vi "LaserMachiningMC.vi"() -> ()   [LabVIEW 2009]
uses:
  <vilib>/Utility/SMTP/NI_SMTPEmail.lvlib
panel:
  in  "Tab Control":T1(tab)
  in  "Ring":u16(ring) items=["Machine Mode", "Write TRJs", "Do nothing"]
  in  "Pause Machining":bool
  in  "Machine this Element":bool
  in  "Create Element":bool
  in  "Make new Element":u16(ring)=5 items=["Make new Capillary", "Make new Slot", "Make new Jet", "Make new Elektrode Hole", "Create Origin Cross"]
  in  "Delete Item":bool
  in  "Element-Liste":i32[](listbox)
  in  "OK":bool
  out "Element Description":variant
  out "Element Name":string
  in  "Abort Machining":bool
  in  "Write to XPS":bool
  in  "Mail notification recipients":string[](array[string])=["ckoschitzki@lbl.gov"]
  out "Current State":string
  in  "Measured origin x,y":dbl[](array[numeric])=[0.83, 0.79]
  in  "Ture: Z home serch 2":bool
  in  "Ture: XY home serch":bool
  in  "Ture: execute trj":bool
  in  "Z Axis Position(S) (units)":dbl=13.8 format="%.6f"
  in  "Ablation Rate":dbl
  out "Move Lens":bool
  in  "XY Line Arc Trajectory":T2={"Velocity (units/s)"=2.0, "Acceleration (unts/s2)"=20.0, "Number of times of execution"=1} {"Acceleration (unts/s2)" format="%.6f"; "Velocity (units/s)" format="%.6f"; "Number of times of execution" format="%.6f"}
  in  "Group Name":string="XY"
  in  "IP address":string="192.168.0.254"
  in  "GPIO Name (DO)":string="GPIO4.DO"
  in  "SingleAxis Group  Name":string="S"
  out "error out":errorcluster
  out "XPS error out":errorcluster
  out "XPS error out(FTP put)":errorcluster
  out "invalid recipients":string[](array[string])
  out "connection ID out":T3
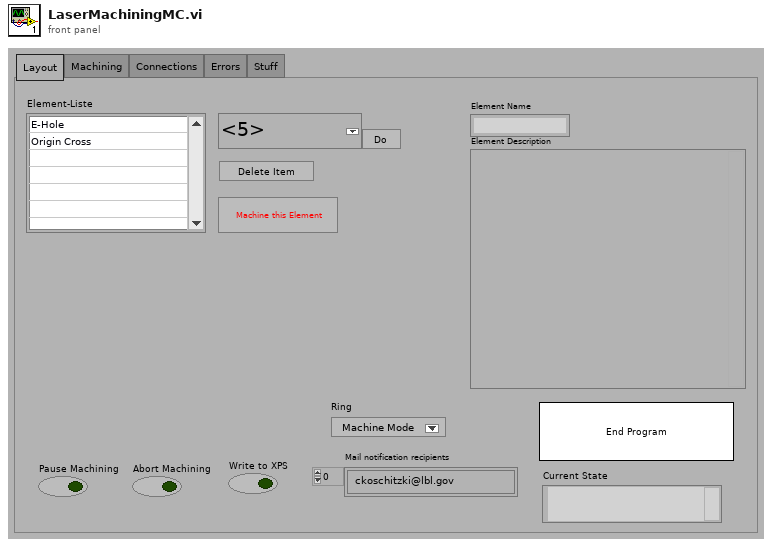
[diagram p1: front panel]
types:
  T1 = enum32{"Layout", "Machining", "Connections", "Errors", "Stuff"}
  T2 = cluster{"Velocity (units/s)":dbl, "Acceleration (unts/s2)":dbl, "Number of times of execution":i32}
  T3 = cluster{"connection TCP":refnum<k5>, "LogTo File":bool, "Log File refnum":refnum<file>, "no error if error log":bool}
  T4 = enum32{"invalid app kind", "Development System", "Run Time System", "Student Edition", "Embedded LabVIEW", "Evaluation", "Custom"}
  T5 = enum32{"Invalid", "Standard", "Closed", "Hidden", "Minimized", "Maximized"}
  T6 = cluster{"Core":cluster{"Current VI Reference":refnum<vi>, "Close Panel on Exit?":bool}, "Elements List":cluster{"Element name":string, "Type":i32, "Layer per L-Move":i32, "Variant":variant}[], "Elements available":cluster{"path":path, "Elements Name":string, "Type":i32}[], "TRJ Cluster":cluster{"TRJs":path[], "size(s)":i32, "Start Point":dbl[][]}, "Start Point":dbl[][], "Additional Stuff":i32, "connection ID":cluster{"connection TCP":refnum<k5>, "LogTo File":bool, "Log File refnum":refnum<file>, "no error if error log":bool}, "IP address":string, "Current TRJ":i32, "GPIO Name (DO) ":string, "XPS error":errorcluster, "Group Name":string, "Measured origin x,y":dbl[], "XY Line Arc Trajectory":cluster{"Velocity (units/s)":dbl, "Acceleration (unts/s2)":dbl, "Number of times of execution":i32}, "Actual Element":cluster{"Element name":string, "Type":i32, "Layer per L-Move":i32, "Variant":variant}}
  T7 = cluster{"Element name":string, "Type":i32, "Layer per L-Move":i32, "Variant":variant}[]
  T8 = cluster{"Element name":string, "Type":i32, "Layer per L-Move":i32, "Variant":variant}
  T9 = cluster{"TRJs":path[], "size(s)":i32, "Start Point":dbl[][]}
  T10 = cluster{"Current VI Reference":refnum<vi>, "Close Panel on Exit?":bool}
  T11 = cluster{"path":path, "Elements Name":string, "Type":i32}[]
  T12 = cluster{"path":path, "Elements Name":string, "Type":i32}
  T13 = cluster{"trj file path(1)":path[], "size(s)":i32, dbl[][]}
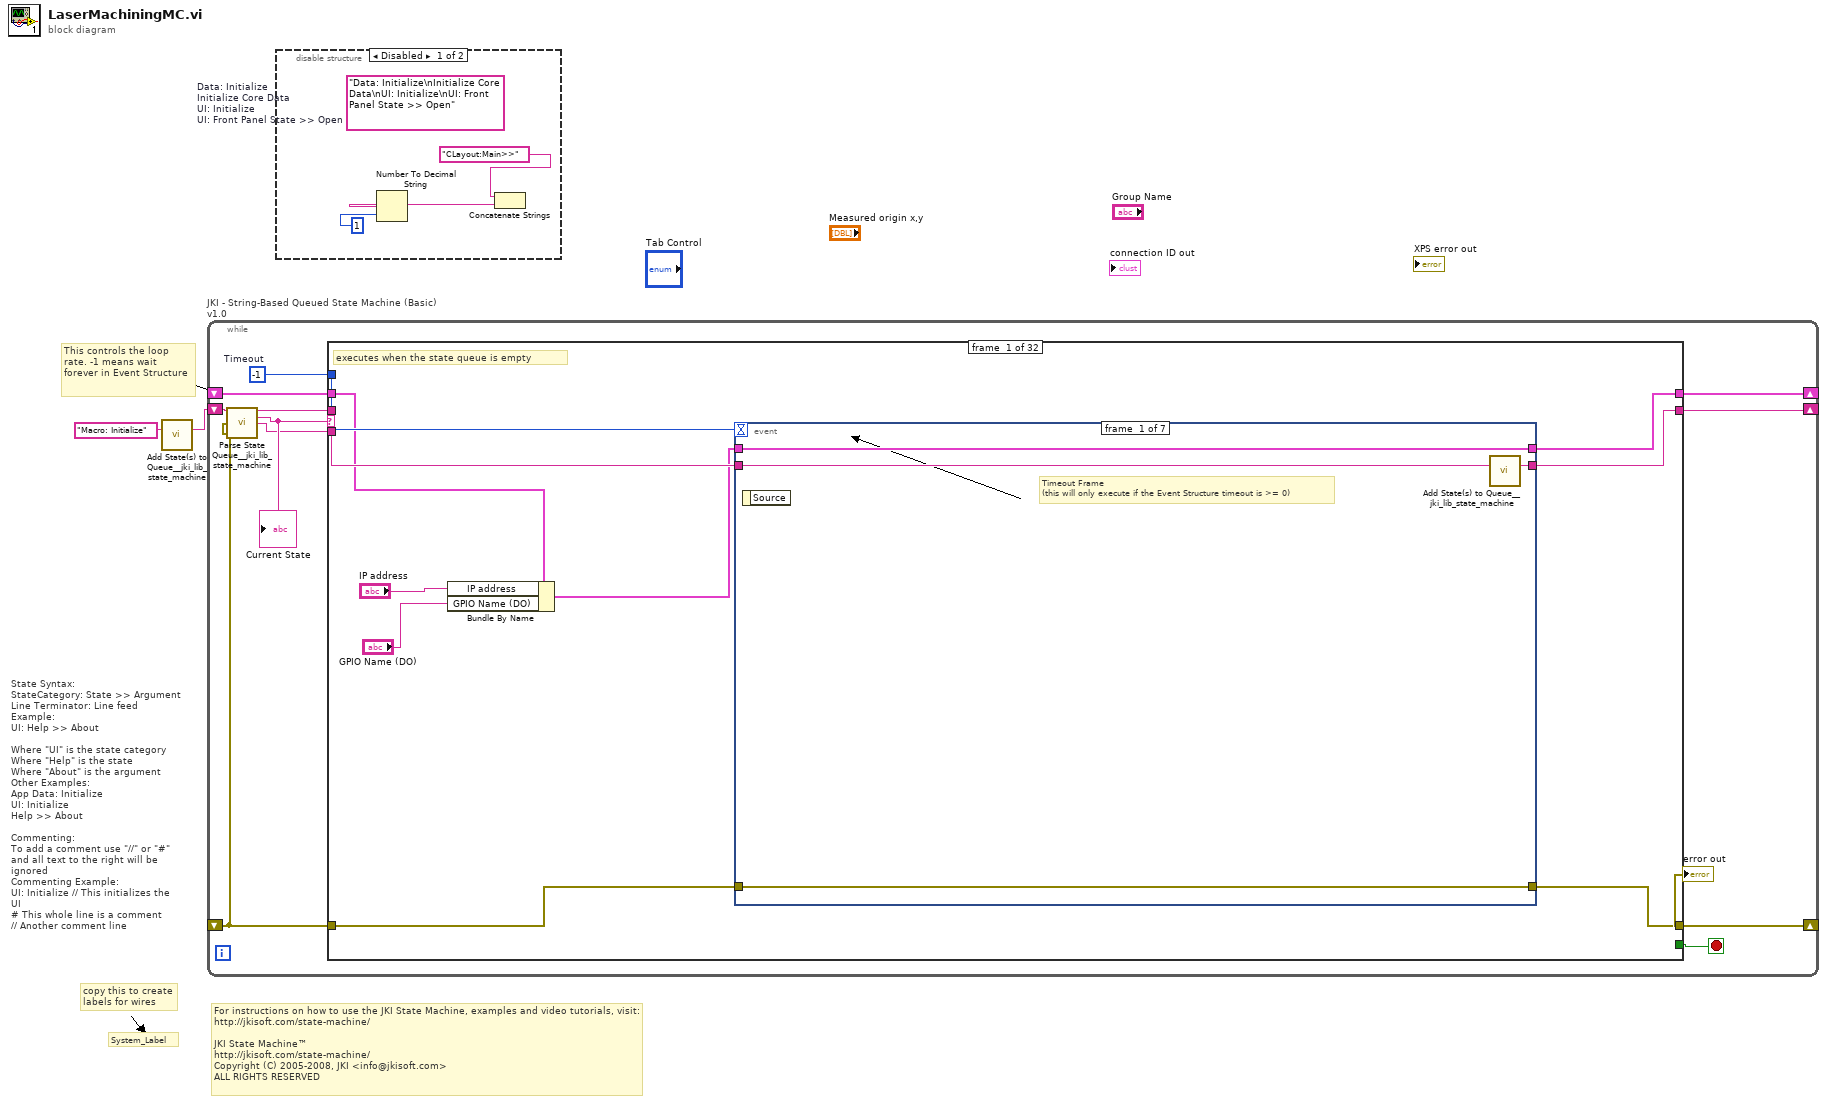
[diagram p0: block diagram]
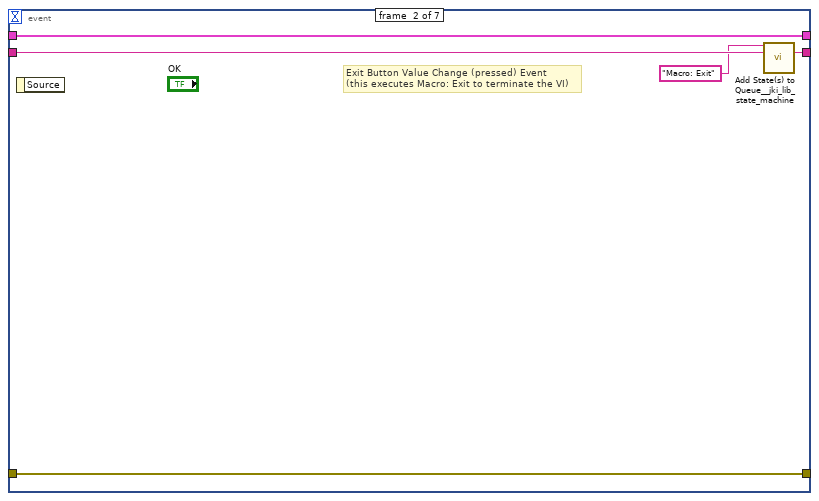
[diagram p3: hidden frame]
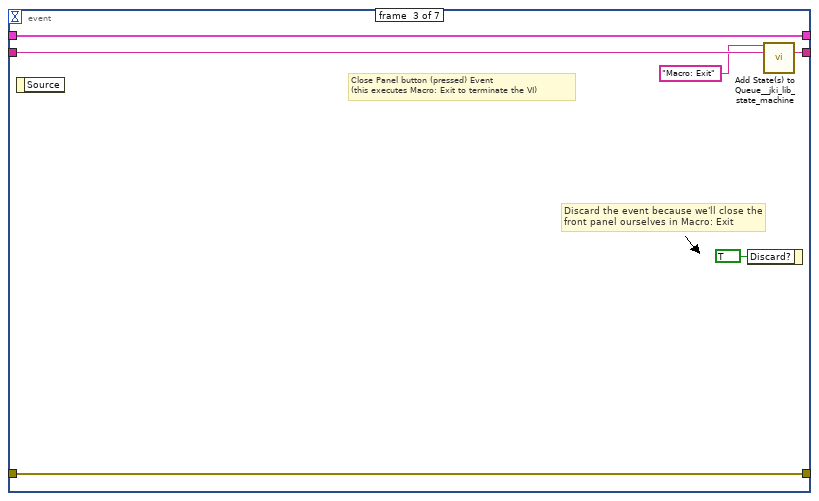
[diagram p4: hidden frame]
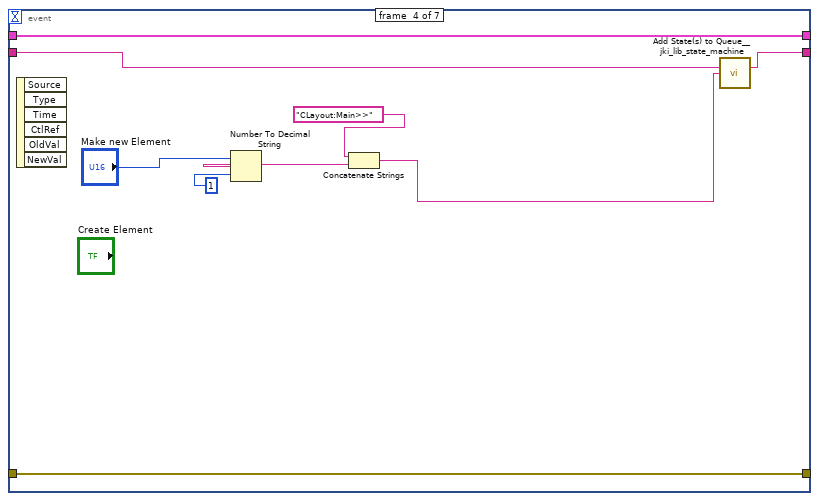
[diagram p5: hidden frame]
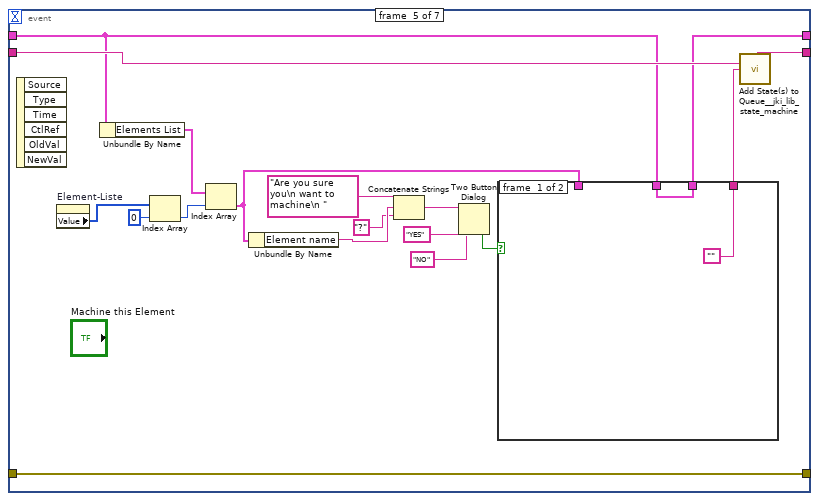
[diagram p6: hidden frame]
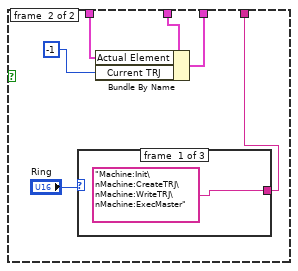
[diagram p7: hidden frame]
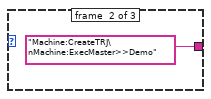
[diagram p8: hidden frame]
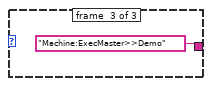
[diagram p9: hidden frame]
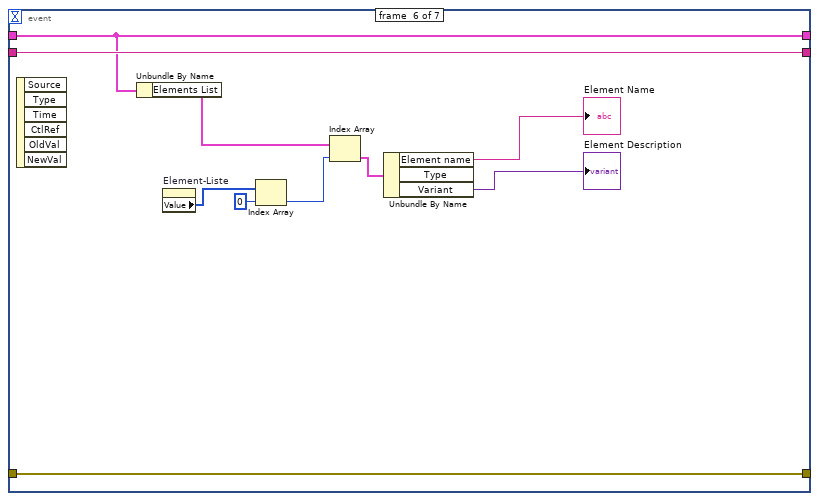
[diagram p10: hidden frame]
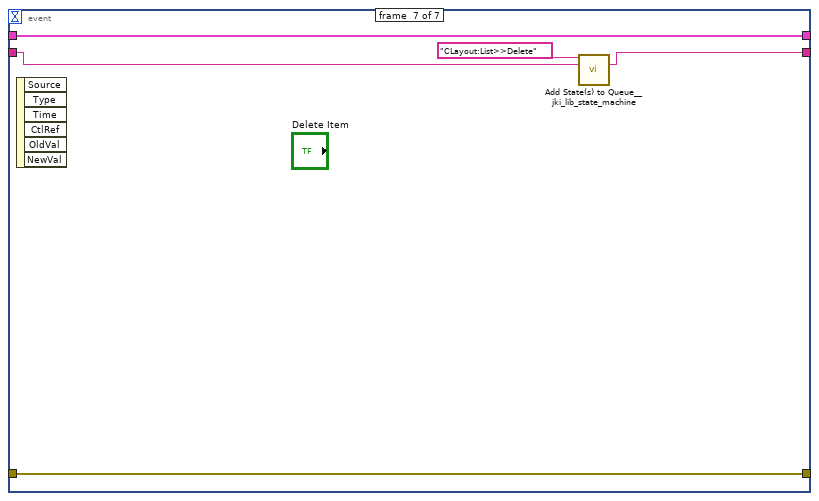
[diagram p11: hidden frame]
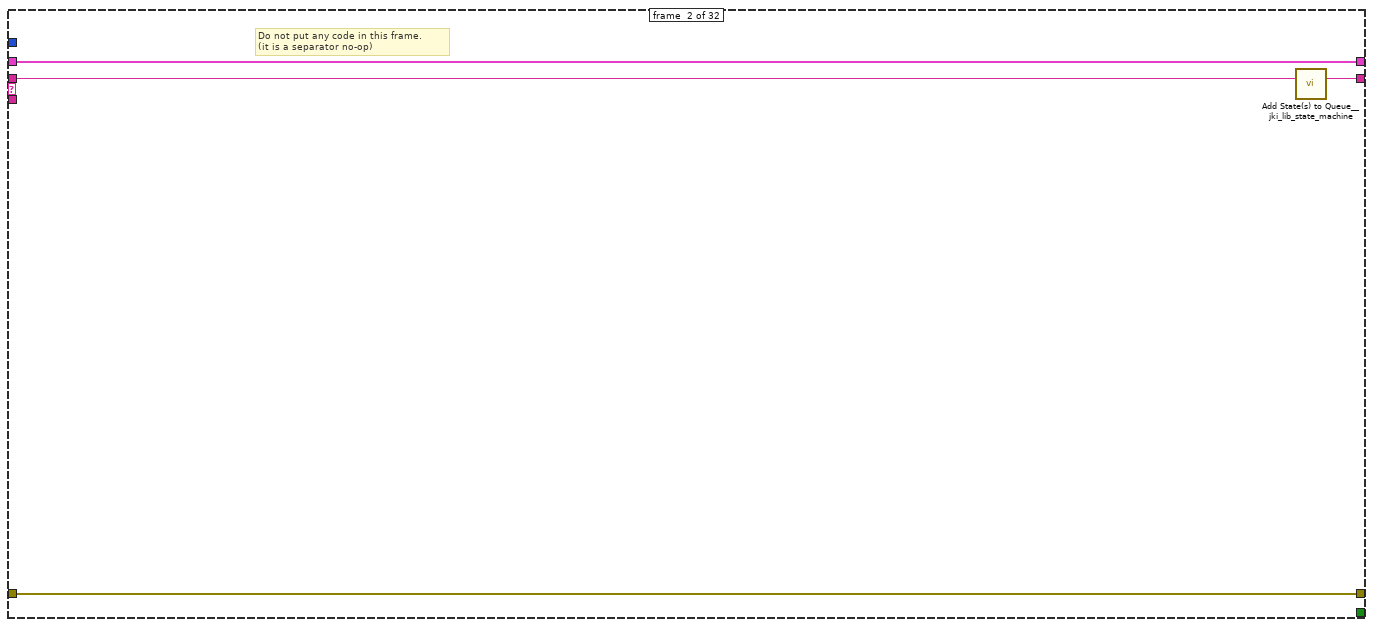
[diagram p12: hidden frame]
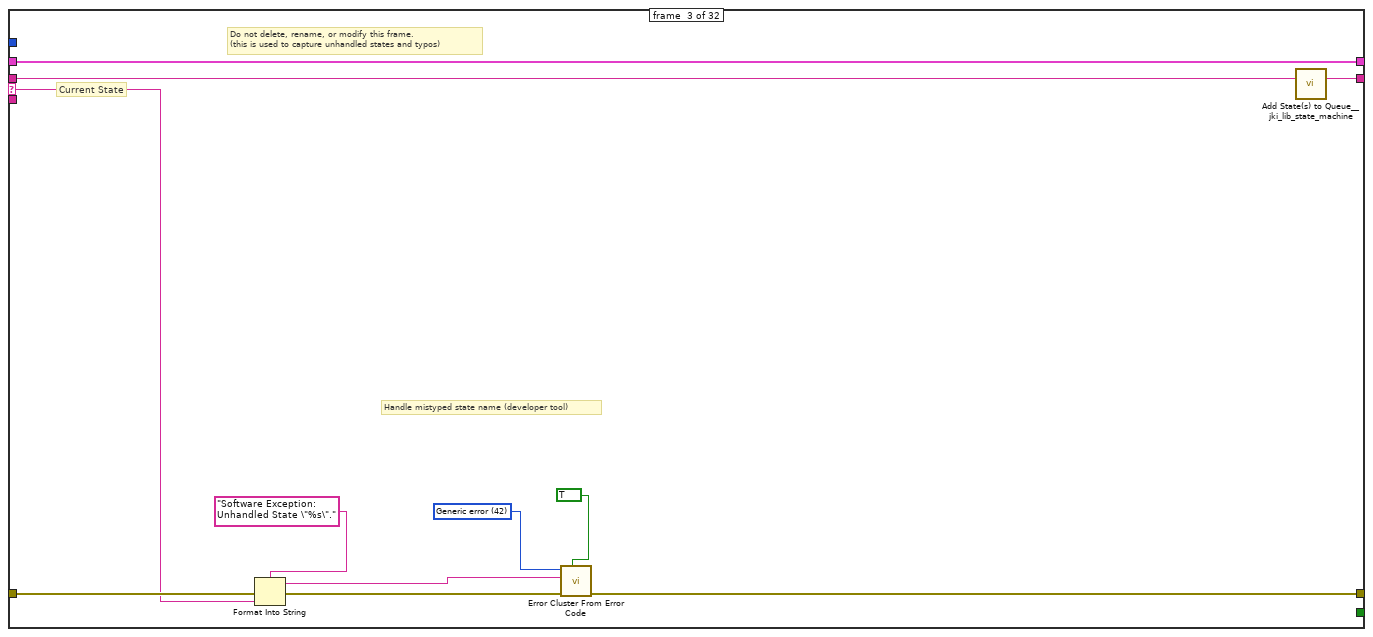
[diagram p13: hidden frame]
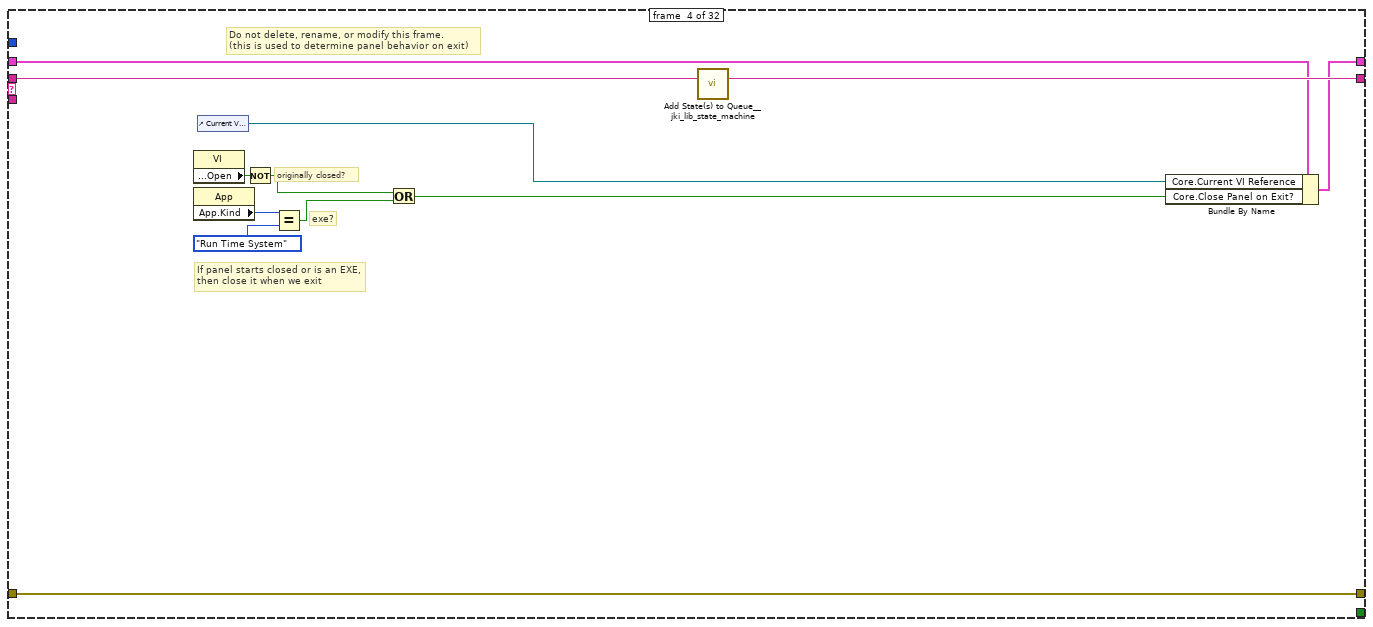
[diagram p14: hidden frame]
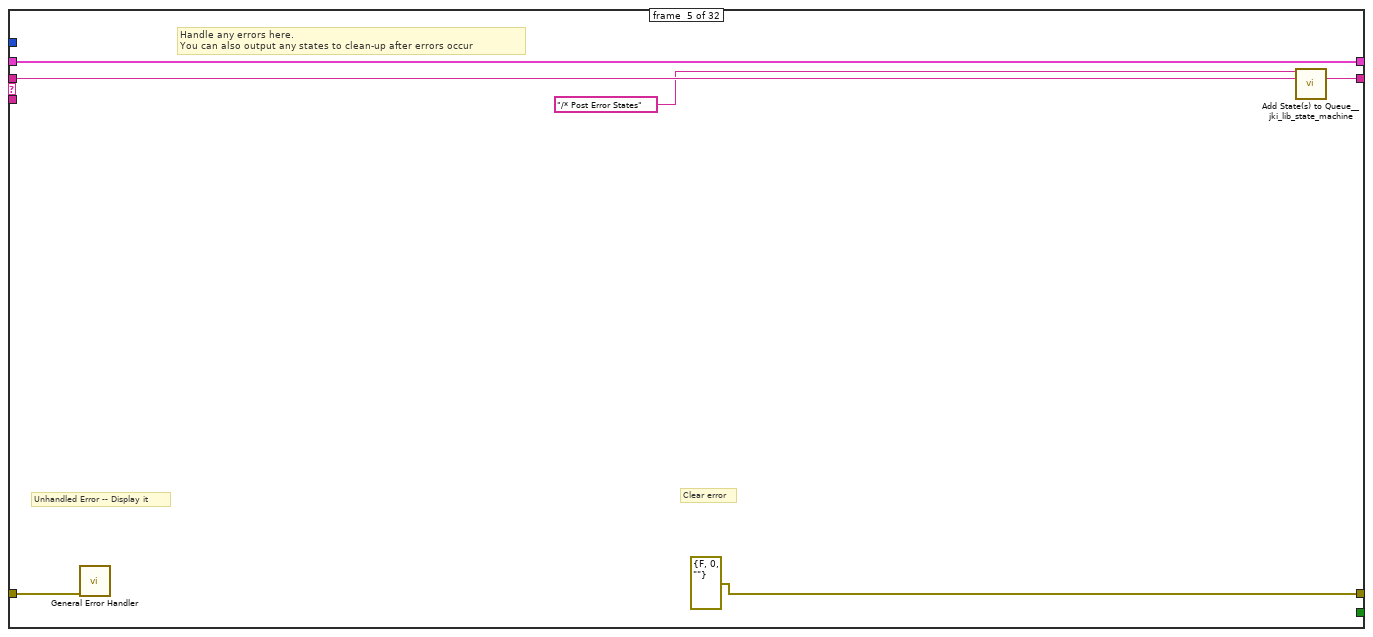
[diagram p15: hidden frame]
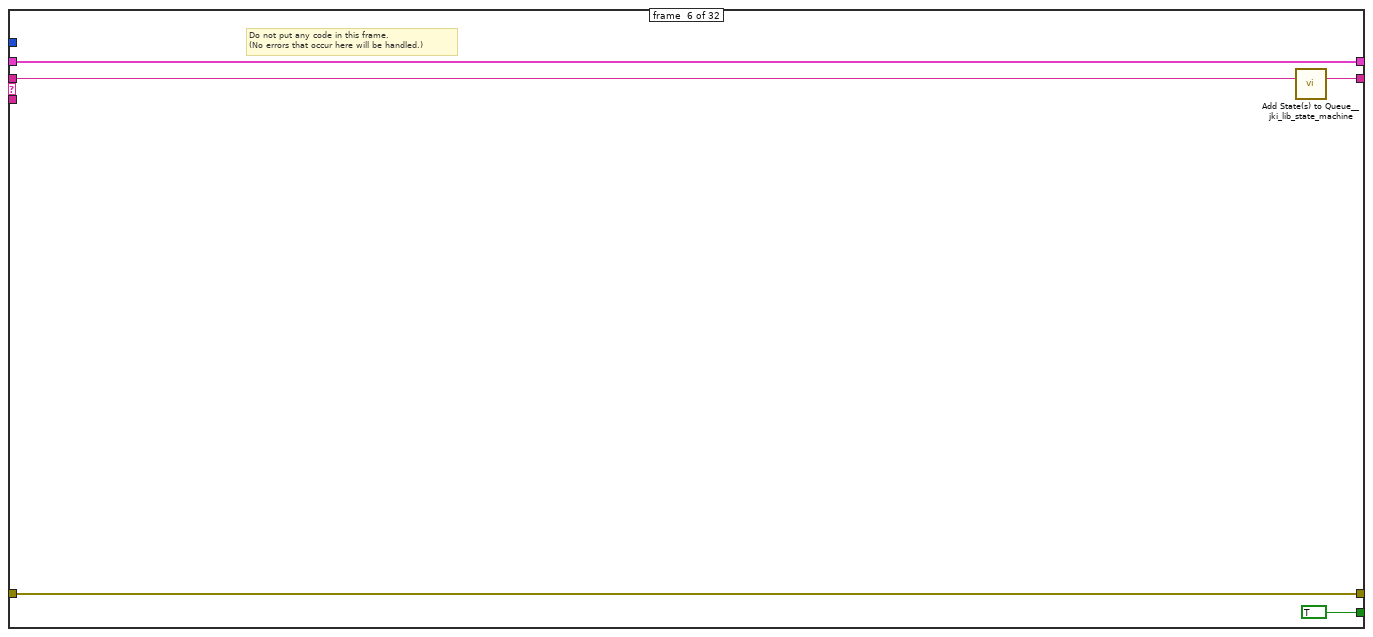
[diagram p16: hidden frame]
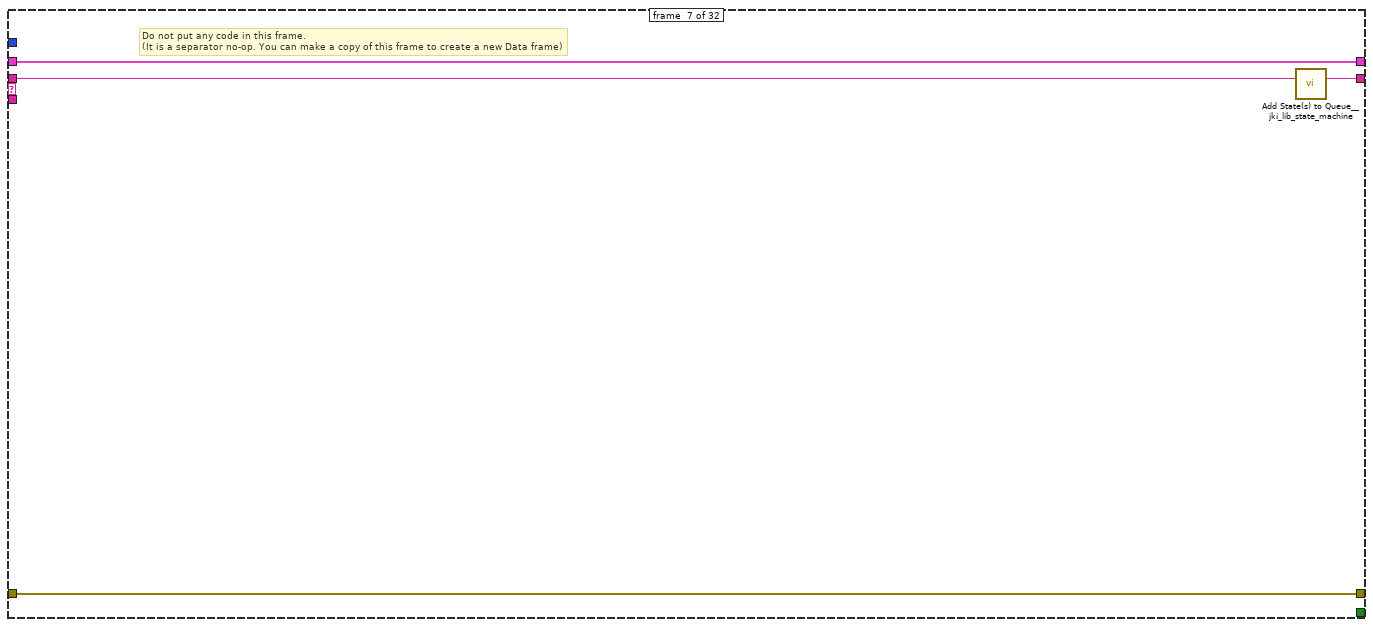
[diagram p17: hidden frame]
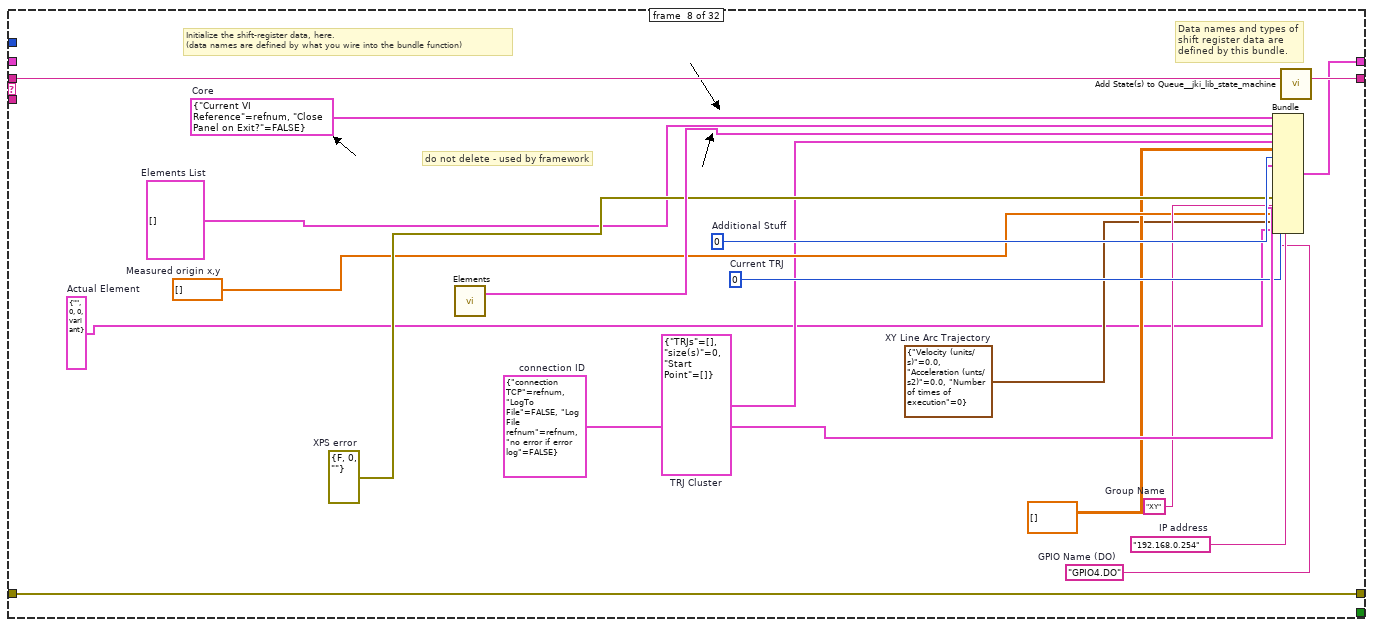
[diagram p18: hidden frame]
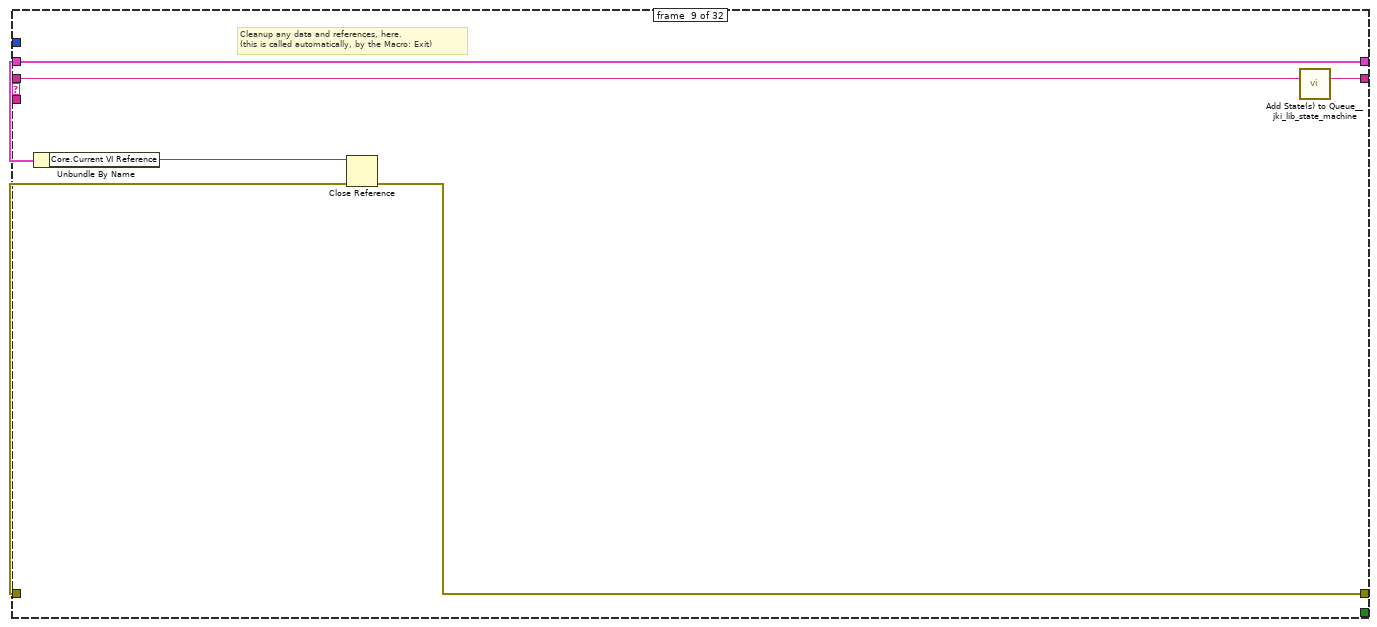
[diagram p19: hidden frame]
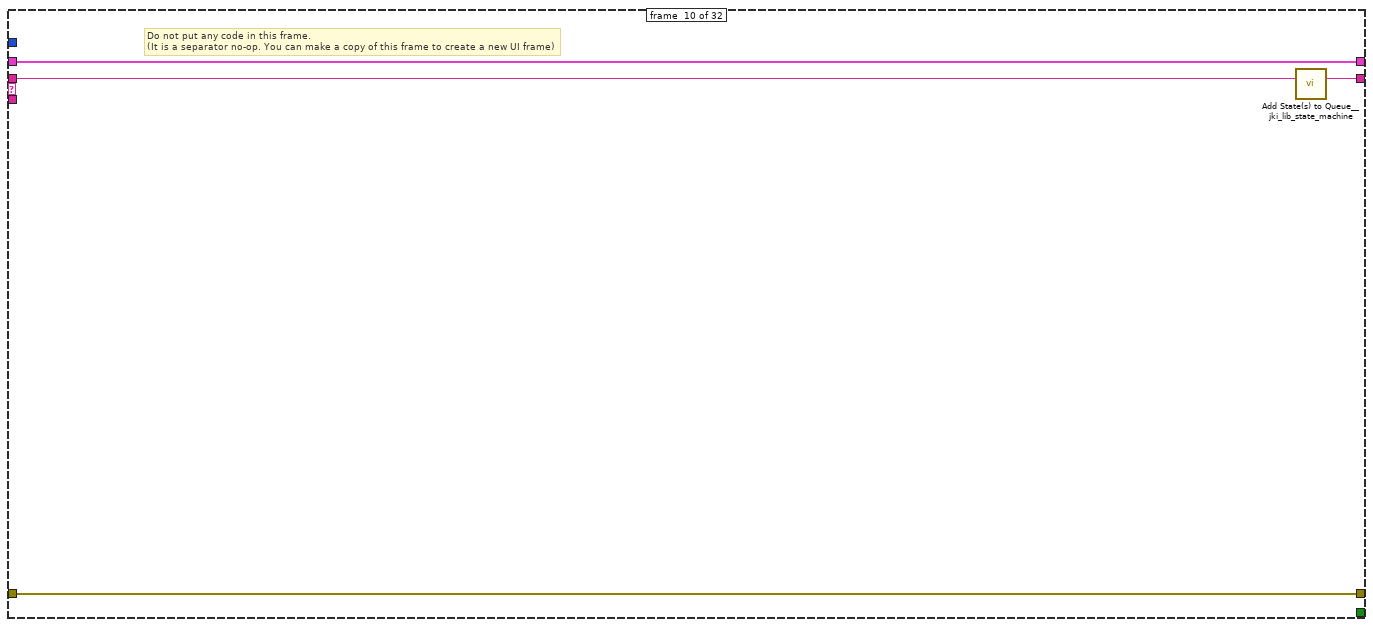
[diagram p20: hidden frame]
diagram:
  # "For instructions on how to use the JKI State Machine, examples and video tutorials, visit:\nhttp://jkisoft.com/state-machine/\n\nJKI State Machine™\nhttp://jkisoft.com/state-machine/\nCopyright (C) 2005-2008, JKI <info@jkisoft.com>\nALL RIGHTS RESERVED"
  # "State Syntax:\nStateCategory: State >> Argument\nLine Terminator: Line feed\nExample:\nUI: Help >> About\n\nWhere \"UI\" is the state category\nWhere \"Help\" is the state\nWhere \"About\" is the argument\nOther Examples:\nApp Data: Initialize\nUI: Initialize\nHelp >> About\n\nCommenting:\nTo add a comment use \"//\" or \"#\" and all text to the right will be ignored\nCommenting Example:\nUI: Initialize // This initializes the UI\n# This whole line is a comment\n// Another comment line"
  # "copy this to create labels for wires"
  # "This controls the loop rate. -1 means wait forever in Event Structure"
  # "System_Label"
  n1 = call <vilib>:"Add State(s) to Queue__jki_lib_state_machine.vi"("State(s) in (\"\")"="Macro: Initialize") -> ("States Out"=w2:string)  [unwired: 14 in]
  n2 = while "JKI - String-Based Queued State Machine (Basic) v1.0" {
    shift-right: [w4] -> _
    shift-left: _ -> [w7]
    shift-right: [w3] -> _
    shift-left: _ -> [w5]
    shift-right: [w9] -> _
    shift-left: w2 -> [w10]
    stop <- w8 stop-if-true
    w6 = -1  # Timeout
    # "Template Copyright © 2008 JKI - http://jkisoft.com/state-machine"
    n3 = call <vilib>:"Parse State Queue__jki_lib_state_machine.vi"("State Queue"=w10, "Error In (no error)"=w5) -> ("Remaining States"=w12:string, "Current State"=w13:string, "Arguments"=w11:string)  [unwired: 11 in]
    "Current State" <- w13
    n4 = case shown="\"CLayout:Main\"" w13 {
      selector: w13 -> [_ _ w96 _ _ _ _ _ _ _ _ _ _ _ _ _ _ _ _ _ _ _ _ _ _ _ _ _ _ _ _ _]
      tunnel: w12 -> [w23 w95 w100 w118 w124 w129 w133 w152 w158 w162 w172 w178 w189 w213 w218 w228 w232 w235 w270 w307 w319 w334 w349 w426 w433 w489 w504 w531 w532 w558 w579 w586]
      tunnel: w11 -> [_ _ _ _ _ _ _ _ _ _ _ w173 w184 _ _ _ _ w236 w265 _ w313 _ w335 _ _ w492 _ _ w539 _ _ _]
      tunnel: w7 -> [w17 w92 w98 w108 w121 w127 w130 _ w154 w159 w169 w176 w183 w210 w215 w219 w229 w238 w264 w304 w317 w331 w339 w424 w431 w490 w505 w528 w537 w557 w578 w583]
      tunnel: [w21 w93 w102 w116 errorcluster {"status"=FALSE, "code"=0, "source"=""} ("error out") w126 w131 w150 w155 w160 w163 w174 w186 w211 w216 w226 w230 w237 w267 w305 w311 w332 w347 w408 w435 w487 w501 w529 w540 w549 w580 w584] -> w3
      tunnel: w5 -> [w20 w93 w101 w116 w120 w126 w131 w150 w156 w160 w166 w175 w187 w211 w216 w226 w230 w237 w268 w305 w312 w332 w347 w409 w438 w488 w502 w530 w541 w550 w581 w584]
      tunnel: [w22 w94 w99 w117 w123 w128 w132 w151 w157 w161 w171 w177 w188 w212 w217 w227 w231 w234 w269 w306 w318 w333 w348 w426 w433 w489 w504 w531 w532 w558 w579 w585] -> w9
      tunnel: [_ _ _ _ _ TRUE _ _ _ _ _ _ _ _ _ _ _ _ _ _ _ _ _ _ _ _ _ _ _ _ _ _] -> w8
      tunnel: [w19 w92 w98 w107 w121 w127 w130 w148 w154 w159 w169 w176 w183 w210 w215 w219 w229 w233 w266 w304 w317 w331 w338 w425 w429 w490 w505 w527 w533 w555 w578 w583] -> w4
      tunnel: w6 -> [w18 _ _ _ _ _ _ _ _ _ _ _ _ _ _ _ _ _ _ _ _ _ _ _ _ _ _ _ _ _ _ _]
      frame #0 {
        # "executes when the state queue is empty"
        n5 = Bundle By Name(cluster=w17, "IP address"="IP address", "GPIO Name (DO)"="GPIO Name (DO)") -> (w16:T6)
        n6 = event shown="[4] \"Machine this Element\": Value Change" {
          selector: _ -> [_ _ _ _ _ _ _]
          dyn-events: _ -> [_ _ _ _ _ _ _]
          timeout: w18 -> [_ _ _ _ _ _ _]
          tunnel: w23 -> [w27 w32 w38 w46 w64 w86 w90]
          tunnel: [w26 w31 w37 w45 w63 w86 w89] -> w22
          tunnel: w16 -> [w24 w29 w35 w40 w51 w85 w91]
          tunnel: [w25 w30 w36 w47 w65 w84 w87] -> w21
          tunnel: w20 -> [w25 w30 w36 w47 w65 w84 w87]
          tunnel: [w24 w29 w35 w40 w50 w85 w91] -> w19
          event #0 {
            # "Timeout Frame\n(this will only execute if the Event Structure timeout is >= 0)"
            n7 = event-data() -> ()  [unwired: 1 in, 1 out]
            n8 = call <vilib>:"Add State(s) to Queue__jki_lib_state_machine.vi"("State(s) in (\"\")"=w27) -> ("States Out"=w26:string)  [unwired: 14 in]
          }
          event #1 {
            # "Exit Button Value Change (pressed) Event\n(this executes Macro: Exit to terminate the VI)"
            n9 = event-data() -> ()  [unwired: 1 in, 1 out]
            n10 = call <vilib>:"Add State(s) to Queue__jki_lib_state_machine.vi"("State(s) in Front (\"\")"="Macro: Exit", "State(s) in (\"\")"=w32) -> ("States Out"=w31:string)  [unwired: 13 in]
          }
          event #2 {
            # "Discard the event because we'll close the front panel ourselves in Macro: Exit"
            # "Close Panel button (pressed) Event\n(this executes Macro: Exit to terminate the VI)"
            n11 = event-data() -> ()  [unwired: 1 in, 1 out]
            n12 = event-data("Discard?"=TRUE) -> ()  [unwired: 1 in, 1 out]
            n13 = call <vilib>:"Add State(s) to Queue__jki_lib_state_machine.vi"("State(s) in Front (\"\")"="Macro: Exit", "State(s) in (\"\")"=w38) -> ("States Out"=w37:string)  [unwired: 13 in]
          }
          event #3 {
            n14 = event-data() -> ()  [unwired: 1 in, 6 out]
            n15 = Number To Decimal String(number="Make new Element", width (-)=i16 1) -> (decimal integer string=w42:string)
            n16 = Concatenate Strings("CLayout:Main>>" ("State(s) in Front (\"\")"), w42) -> (w39:string)
            n17 = call <vilib>:"Add State(s) to Queue__jki_lib_state_machine.vi"("State(s) in (\"\")"=w46, "State(s) at Back (\"\")"=w39) -> ("States Out"=w45:string)  [unwired: 13 in]
          }
          event #4 {
            n18 = event-data() -> ()  [unwired: 1 in, 6 out]
            n19 = property on="Element-Liste" class="LstBox (strict)"() -> ("Value"=w62:i32[])  [unwired: 2 in, 2 out]
            n20 = Unbundle By Name(w51) -> ("Elements List"=w60:T7)
            n21 = Index Array(array=w62, index=0) -> (element=w59:i32)
            n22 = Index Array(array=w60, index=w59) -> (element=w49:T8)
            n23 = Unbundle By Name(w49) -> ("Element name"=w58:string)
            n24 = Concatenate Strings("Are you sure you\n want to machine\n " ("message"), w58, "?" ("string")) -> (w56:string)
            n25 = Two Button Dialog(message=w56, 1:"NO" ("F button name (\"Cancel\")"), 2:"YES" ("T button name (\"OK\")")) -> (T button?=w52:bool)
            n26 = case shown="True" w52 {
              tunnel: w51 -> [w67 w73]
              tunnel: [w67 w72] -> w50
              tunnel: w49 -> [_ w71]
              tunnel: ["" w68] -> w48
              frame #0 {
              }
              frame #1 {
                n27 = case shown="1" "Ring" {
                  tunnel: ["Machine:Init\nMachine:CreateTRJ\nMachine:WriteTRJ\nMachine:ExecMaster" ("message") "Machine:CreateTRJ\nMachine:ExecMaster>>Demo" ("message") "Machine:ExecMaster>>Demo" ("message")] -> w68
                  frame #0 {
                  }
                  frame #1 {
                  }
                  frame #2 {
                  }
                }
                n28 = Bundle By Name(cluster=w73, "Actual Element"=w71, "Current TRJ"=-1) -> (w72:T6)
              }
            }
            n29 = call <vilib>:"Add State(s) to Queue__jki_lib_state_machine.vi"("State(s) in (\"\")"=w64, "State(s) at Back (\"\")"=w48) -> ("States Out"=w63:string)  [unwired: 13 in]
          }
          event #5 {
            n30 = event-data() -> ()  [unwired: 1 in, 6 out]
            n31 = Unbundle By Name(w85) -> ("Elements List"=w80:T7)
            n32 = property on="Element-Liste" class="LstBox (strict)"() -> ("Value"=w83:i32[])  [unwired: 2 in, 2 out]
            n33 = Index Array(array=w83, index=0) -> (element=w81:i32)
            n34 = Index Array(array=w80, index=w81) -> (element=w79:T8)
            n35 = Unbundle By Name(w79) -> ("Element name"=→"Element Name":string, "Variant"=→"Element Description":variant)  [unwired: 1 out]
          }
          event #6 {
            n36 = event-data() -> ()  [unwired: 1 in, 6 out]
            n37 = call <vilib>:"Add State(s) to Queue__jki_lib_state_machine.vi"("State(s) in Front (\"\")"="CLayout:List>>Delete" ("State(s) in Front (\"\")"), "State(s) in (\"\")"=w90) -> ("States Out"=w89:string)  [unwired: 13 in]
          }
        }
      }
      frame #1 {
        # "Do not put any code in this frame.\n(it is a separator no-op)"
        n38 = call <vilib>:"Add State(s) to Queue__jki_lib_state_machine.vi"("State(s) in (\"\")"=w95) -> ("States Out"=w94:string)  [unwired: 14 in]
      }
      frame #2 {
        w105 = 42 items=["No error", "Argument error", "Memory is full", "Out of zone", "End of file", "File already open", "Generic file I/O error", "File not found", "File permission error", "Disk is full", "Duplicate path", "Too many files open", "System feature not enabled", "Resource file not found", "Cannot add resource", "Resource not found", "Image not found", "Image memory error", "Pen does not exist", "Config type invalid", "Config token not found", "Config parse error", "Config memory error", "Bad external code format", "Bad external code offset", "External code not present", "Null window", "Destroy window error", "Null menu", "Print aborted", "Bad print record", "Print driver error", "Windows error during printing", "Memory error during printing", "Print dialog error", "Generic print error", "Invalid device refnum", "Device not found", "Device parameter error", "Device unit error", "Cannot open device", "Device call aborted", "Generic error", "Cancelled by user", "Object ID too low", "Object ID too high", "Object not in heap", "Unknown heap", "Unknown object (invalid DefProc)", "Unknown object (DefProc not in table)", "Message out of range", "Invalid (null) method", "Unknown message", "Manager call not supported", "Bad address", "Network operation in progress", "Network operation timed out", "Connection is busy", "Network attribute not supported", "Network error", "Address in use", "System out of memory", "Connection aborted", "Connection refused", "Not connected", "Already connected", "Connection closed", "Initialization error (interapplication manager)", "Bad occurrence", "Wait on unbound occurrence handler", "Occurrence queue overflow", "Datalog type conflict", "Unused", "Unrecognized type (interapplication manager)", "Memory corrupt", "Failed to make temporary DLL", "Old CIN version", "Drag socket not found", "Failed to load drop-object", "Failed to register OLE object", "Failed to release OLE object", "Format specifier type mismatch", "Unknown format specifier", "Too few format specifiers", "Too many format specifiers", "Scan failed", "Newer CIN version", "Error converting to variant", "Runtime menu error", "Password tampered", "Variant attribute not found", "Incompatible variant data type", "Event data is not available", "Event Store is not present", "Occurrence is not found", "Event Queue is not created", "Event info is not available", "Refnum passed is NULL", "Error retrieving Class GUID", "Error retrieving CoClass GUID", "Error retrieving TypeLib GUID.", "Bad built application magic bytes.", "Specific driver is different from the specific driver associated with the Logical Name.", "There is no session opened to the class driver.", "Max Error", "MAX - Error with config objects", "MAX - Error loading configuration", "MAX - Group not supported"]
        # "Current State"
        # "Do not delete, rename, or modify this frame.\n(this is used to capture unhandled states and typos)"
        # "Handle mistyped state name (developer tool)"
        n39 = Format Into String(format string="Software Exception: Unhandled State \"%s\"." ("message"), error in=w101, w96) -> (resulting string=w104:string, error out=w103:errorcluster)  [unwired: 1 in]
        n40 = call <vilib>:"Error Cluster From Error Code.vi"("show call chain? (False)"=TRUE, "error in (no error)"=w103, "error message (\"\")"=w104, "error code (0)"=w105) -> ("error out"=w102:errorcluster)  [unwired: 5 in]
        n41 = call <vilib>:"Add State(s) to Queue__jki_lib_state_machine.vi"("State(s) in (\"\")"=w100) -> ("States Out"=w99:string)  [unwired: 14 in]
      }
      frame #3 {
        # "Do not delete, rename, or modify this frame.\n(this is used to determine panel behavior on exit)"
        # "originally closed?"
        # "exe?"
        # "If panel starts closed or is an EXE, then close it when we exit"
        n42 = property class="VI"() -> ("Front Panel.Open"=w115:bool)  [unwired: 2 in, 2 out]
        n43 = property class="App"() -> ("App.Kind"=w114:T4)  [unwired: 2 in, 2 out]
        n44 = control-ref of="Current VI Reference"() -> (w109:refnum<vi>)
        n45 = Not(x=w115) -> (.not. x?=w112:bool)
        n46 = Equal?(x=w114, y=T4."Run Time System" ("Application:Kind")) -> (x = y?=w111:bool)
        n47 = Or(x=w112, y=w111) -> (x .or. y?=w110:bool)
        n48 = call <vilib>:"Add State(s) to Queue__jki_lib_state_machine.vi"("State(s) in (\"\")"=w118) -> ("States Out"=w117:string)  [unwired: 14 in]
        n49 = Bundle By Name(cluster=w108, "Core.Current VI Reference"=w109, "Core.Close Panel on Exit?"=w110) -> (w107:T6)
      }
      frame #4 {
        # "Unhandled Error -- Display it"
        # "Handle any errors here.\nYou can also output any states to clean-up after errors occur"
        # "Clear error"
        n50 = call <vilib>:"General Error Handler.vi"("error in (no error)"=w120) -> ()  [unwired: 10 in, 5 out]
        n51 = call <vilib>:"Add State(s) to Queue__jki_lib_state_machine.vi"("State(s) in Front (\"\")"="/* Post Error States", "State(s) in (\"\")"=w124) -> ("States Out"=w123:string)  [unwired: 13 in]
      }
      frame #5 {
        # "Do not put any code in this frame.\n(No errors that occur here will be handled.)"
        n52 = call <vilib>:"Add State(s) to Queue__jki_lib_state_machine.vi"("State(s) in (\"\")"=w129) -> ("States Out"=w128:string)  [unwired: 14 in]
      }
      frame #6 {
        # "Do not put any code in this frame.\n(It is a separator no-op. You can make a copy of this frame to create a new Data frame)"
        n53 = call <vilib>:"Add State(s) to Queue__jki_lib_state_machine.vi"("State(s) in (\"\")"=w133) -> ("States Out"=w132:string)  [unwired: 14 in]
      }
      frame #7 {
        w134 = T8 {"Element name"="", "Type"=0, "Layer per L-Move"=0, "Variant"=variant}  # Actual Element
        w135 = T7 []  # Elements List
        w136 = T2 {"Velocity (units/s)"=0.0, "Acceleration (unts/s2)"=0.0, "Number of times of execution"=0}  # XY Line Arc Trajectory
        w137 = T9 {"TRJs"=[], "size(s)"=0, "Start Point"=[]}  # TRJ Cluster
        w139 = dbl[] []  # Measured origin x,y
        w140 = "XY"  # Group Name
        w141 = errorcluster {"status"=FALSE, "code"=0, "source"=""}  # XPS error
        w142 = "GPIO4.DO"  # GPIO Name (DO)
        w143 = 0  # Current TRJ
        w144 = "192.168.0.254"  # IP address
        w145 = T3 {"connection TCP"=refnum, "LogTo File"=FALSE, "Log File refnum"=refnum, "no error if error log"=FALSE}  # connection ID
        w146 = 0  # Additional Stuff
        w149 = T10 {"Current VI Reference"=refnum, "Close Panel on Exit?"=FALSE}  # Core
        # "do not delete - used by framework"
        # "Data names and types of shift register data are defined by this bundle."
        # "Initialize the shift-register data, here.\n(data names are defined by what you wire into the bundle function)"
        n54 = call "Elements.vi"() -> ("Elements available"=w147:T11)  [unwired: 2 in]
        n55 = Bundle("Core"=w149, "Elements List"=w135, "Elements available"=w147, "TRJ Cluster"=w137, "Start Point"=dbl[][] [], "Additional Stuff"=w146, "connection ID"=w145, "IP address"=w144, "Current TRJ"=w143, "GPIO Name (DO)"=w142, "XPS error"=w141, "Group Name"=w140, "Measured origin x,y"=w139, "XY Line Arc Trajectory"=w136, "Actual Element"=w134) -> (w148:T6)  [unwired: 1 in]
        n56 = call <vilib>:"Add State(s) to Queue__jki_lib_state_machine.vi"("State(s) in (\"\")"=w152) -> ("States Out"=w151:string)  [unwired: 14 in]
      }
      frame #8 {
        # "Cleanup any data and references, here.\n(this is called automatically, by the Macro: Exit)"
        n57 = Unbundle By Name(w154) -> ("Core.Current VI Reference"=w153:refnum<vi>)
        n58 = Close Reference(reference=w153, error in (no error)=w156) -> (error out=w155:errorcluster)
        n59 = call <vilib>:"Add State(s) to Queue__jki_lib_state_machine.vi"("State(s) in (\"\")"=w158) -> ("States Out"=w157:string)  [unwired: 14 in]
      }
      frame #9 {
        # "Do not put any code in this frame.\n(It is a separator no-op. You can make a copy of this frame to create a new UI frame)"
        n60 = call <vilib>:"Add State(s) to Queue__jki_lib_state_machine.vi"("State(s) in (\"\")"=w162) -> ("States Out"=w161:string)  [unwired: 14 in]
      }
      frame #10 {
        # "Initialize the User Interface, here.\n(this is called automatically, by the Macro: Init)"
        n61 = Unbundle By Name(w169) -> ("Elements available"=w168:T11)
        n62 = call "Init_Ring.vi"("Elements available"=w168) -> ("Array"=w167:cluster{"string":string, i32}[])
        n63 = property on="Make new Element" class="Ring (strict)"(error in=w166, "StringsAndValues[]"=w167) -> (error out=w165:errorcluster)  [unwired: 1 in, 1 out]
        n64 = property on="Make new Element" class="Ring (strict)"(error in=w165, "Value"=0) -> (error out=w163:errorcluster)  [unwired: 1 in, 1 out]
        n65 = call <vilib>:"Add State(s) to Queue__jki_lib_state_machine.vi"("State(s) in (\"\")"=w172, "State(s) at Back (\"\")"="CLayout:List>>Init" ("State(s) at Back (\"\")")) -> ("States Out"=w171:string)  [unwired: 13 in]
      }
      frame #11 {
        # "Argument"
        # "Set and Unset Cursor Busy.\n(Usage: \"UI: Cursor Set >> Busy|Idle\")"
        n66 = case shown="\"Idle\", Default" w173 {
          tunnel: w175 -> [w180 w182]
          tunnel: [w179 w181] -> w174
          frame #0 {
            n67 = call <vilib>:"Unset Busy.vi"("error in (no error)"=w180) -> ("error out"=w179:errorcluster)  [unwired: 10 in]
          }
          frame #1 {
            n68 = call <vilib>:"Set Busy.vi"("error in (no error)"=w182) -> ("error out"=w181:errorcluster)  [unwired: 9 in, 1 out]
          }
        }
        n69 = call <vilib>:"Add State(s) to Queue__jki_lib_state_machine.vi"("State(s) in (\"\")"=w178) -> ("States Out"=w177:string)  [unwired: 14 in]
      }
      frame #12 {
        # "Argument"
        # "Set Front Panel Open or Closed\n(Usage: \"UI: Front Panel State >> Open|Close\")"
        n70 = Unbundle By Name(w183) -> ("Core.Current VI Reference"=w185:refnum<vi>)
        n71 = case shown="\"Open\", Default" w184 {
          tunnel: w187 -> [w193 w204]
          tunnel: [w194 w205] -> w186
          tunnel: w185 -> [_ _]
          frame #0 {
            n72 = property class="VI"(error in=w193) -> (reference out=w191:refnum<vi>, error out=w192:errorcluster, "Front Panel.Open"=w190:bool)  [unwired: 1 in]
            n73 = case shown="False" w190 {
              tunnel: [w197 w200] -> w194
              tunnel: w192 -> [w196 w200]
              tunnel: w191 -> [w195 _]
              frame #0 {
                n74 = invoke class="VI" method="FP.Open"(reference=w195, error in=w196, "Activate"=TRUE, "State"=T5."Standard") -> (error out=w197:errorcluster)  [unwired: 1 in, 4 out]
              }
              frame #1 {
              }
            }
          }
          frame #1 {
            n75 = property class="VI"(error in=w204) -> (reference out=w202:refnum<vi>, error out=w203:errorcluster, "Front Panel.Open"=w201:bool)  [unwired: 1 in]
            n76 = case shown="True" w201 {
              tunnel: [w206 w209] -> w205
              tunnel: w203 -> [w206 w208]
              tunnel: w202 -> [_ w207]
              frame #0 {
              }
              frame #1 {
                n77 = invoke class="VI" method="FP.Close"(reference=w207, error in=w208) -> (error out=w209:errorcluster)  [unwired: 1 in, 2 out]
              }
            }
          }
        }
        n78 = call <vilib>:"Add State(s) to Queue__jki_lib_state_machine.vi"("State(s) in (\"\")"=w189) -> ("States Out"=w188:string)  [unwired: 14 in]
      }
      frame #13 {
        # "Do not put any code in this frame.\n(It is a separator no-op. You can make a copy of this frame to create a new Macro frame)"
        n79 = call <vilib>:"Add State(s) to Queue__jki_lib_state_machine.vi"("State(s) in (\"\")"=w213) -> ("States Out"=w212:string)  [unwired: 14 in]
      }
      frame #14 {
        w214 = "Data: Initialize\nInitialize Core Data\nUI: Initialize\nUI: Front Panel State >> Open"  # Data: Initialize Initialize Core Data UI: Initialize UI: Front Panel State >> Open
        # "Initialization Macro\n(This is called once, when the VI starts)"
        n80 = call <vilib>:"Add State(s) to Queue__jki_lib_state_machine.vi"("State(s) in Front (\"\")"=w214, "State(s) in (\"\")"=w218) -> ("States Out"=w217:string)  [unwired: 13 in]
      }
      frame #15 {
        # "Exit Macro\n(This is called once, when the VI exits)"
        n81 = Unbundle By Name(w219) -> ("Core.Close Panel on Exit?"=w220:bool)
        n82 = Select(t="UI: Front Panel State >> Close", s=w220, f="") -> (s? t:f=w223:string)
        n83 = call <vilib>:"Add State(s) to Queue__jki_lib_state_machine.vi"("State(s) in (\"\")"=w223, "State(s) at Back (\"\")"="Data: Cleanup\nExit") -> ("States Out"=w221:string)  [unwired: 13 in]
        n84 = call <vilib>:"Add State(s) to Queue__jki_lib_state_machine.vi"("State(s) in Front (\"\")"=w221, "State(s) in (\"\")"=w228) -> ("States Out"=w227:string)  [unwired: 13 in]
      }
      frame #16 {
        # "Template Separator\n(You can make a copy of, or modify, this frame)"
        n85 = call <vilib>:"Add State(s) to Queue__jki_lib_state_machine.vi"("State(s) in (\"\")"=w232) -> ("States Out"=w231:string)  [unwired: 14 in]
      }
      frame #17 {
        n86 = case shown="\"Delete\"" w236 {
          tunnel: w238 -> [w239 w241 w247 w258]
          tunnel: w235 -> [w240 w242 w248 w255]
          tunnel: [w240 w242 w248 w254] -> w234
          tunnel: [w239 w241 w247 w256] -> w233
          frame #0 {
          }
          frame #1 {
            n87 = Initialize Array("", 1 ("dimension size")) -> (w244:string[])
            n88 = property on="Element-Liste" class="LstBox (strict)"("Item Names"=w244, "Selection Mode"=1) -> ()  [unwired: 2 in, 2 out]
          }
          frame #2 {
            n89 = Unbundle By Name(w247) -> ("Elements List"=w250:T7)
            n90 = for {
              tunnel: w250 -> [w252] mode=indexing
              tunnel: [w251] -> w249 mode=indexing
              n91 = Unbundle By Name(w252) -> ("Element name"=w251:string)
            }
            n92 = property on="Element-Liste" class="LstBox (strict)"("Item Names"=w249) -> ()  [unwired: 2 in, 2 out]
          }
          frame #3 {
            n93 = Unbundle By Name(w258) -> ("Elements List"=w259:T7)
            n94 = property on="Element-Liste" class="LstBox (strict)"() -> ("Value"=w262:i32[])  [unwired: 2 in, 2 out]
            n95 = Index Array(array=w262, index=0) -> (element=w260:i32)
            n96 = Delete From Array(array=w259, length=1, index=w260) -> (array with subset deleted=w257:T7)  [unwired: 1 out]
            n97 = Bundle By Name(cluster=w258, "Elements List"=w257) -> (w256:T6)
            n98 = call <vilib>:"Add State(s) to Queue__jki_lib_state_machine.vi"("State(s) in Front (\"\")"="CLayout:List>>Update" ("State(s) at Back (\"\")"), "State(s) in (\"\")"=w255) -> ("States Out"=w254:string)  [unwired: 13 in]
          }
        }
      }
      frame #18 {
        n99 = disable-structure shown="Enabled" {
          disable-tunnel: w270 -> [w303 _]
          disable-tunnel: [w302 _] -> w269
          disable-tunnel: w268 -> [w301 _]
          disable-tunnel: [w297 _] -> w267
          disable-tunnel: [w287 _] -> w266
          disable-tunnel: w265 -> [w292 _]
          disable-tunnel: w264 -> [w289 _]
          frame #0 {
            w279 = TRUE ("Execution:Show Front Panel On Call")
            w282 = u16 1 items=["Get Path", "Make Layout"] ("Outputmode")
            # "Erzeugt ein Cap\nDie Daten fuer das Cap werden in die Liste und als aktuelles Element uebernommen"
            n100 = Unbundle By Name(w289) -> ("Elements List"=w290:T7, "Core"=w294:T10, "Elements available"=w291:T11)
            n101 = Unbundle By Name(w294) -> ("Current VI Reference"=w293:refnum<vi>)
            n102 = Fract/Exp String To Number(string=w292, default (0 dbl)=0 ("default (0 DBL)")) -> (number=w285:i32)  [unwired: 2 in, 1 out]
            n103 = property class="VI"(reference=w293, error in=w301, "FP.State"=T5."Hidden" ("Front Panel Window:State")) -> (reference out=w283:refnum<vi>, error out=w299:errorcluster)
            n104 = Index Array(array=w291, index=w285) -> (element=w272:T12)
            n105 = Unbundle By Name(w272) -> ("path"=w271:path)
            n106 = Open VI Reference(type specifier VI Refnum (for type only)=refnum<vi> refnum, vi path=w271, error in (no error)=w299) -> (vi reference=w280:refnum<vi>, error out=w277:errorcluster)  [unwired: 3 in]
            n107 = property class="VI (strict)"(reference=w280, error in=w277, "Exec.ShowFPOnCall"=w279, "Exec.CloseFPAfterCall"=w279) -> (reference out=w274:refnum<vi>, error out=w276:errorcluster)
            n108 = call <vilib>:"Add State(s) to Queue__jki_lib_state_machine.vi"("State(s) in Front (\"\")"="CLayout:List" ("State(s) at Back (\"\")"), "State(s) in (\"\")"=w303) -> ("States Out"=w302:string)  [unwired: 13 in]
            n109 = call-by-ref "Call By Reference Node"(reference=w274, error in=w276, "Outputmode"=w282) -> (reference out=w278:refnum<vi>, error out=w281:errorcluster, "Elements out"=w273:T7)  [unwired: 3 in, 3 out]
            n110 = Array Size(array=w290) -> (size(s)=w296:i32)
            n111 = Insert Into Array(array=w290, index=w296, new element=w273) -> (w288:T7)
            n112 = Close Reference(reference=w278, error in (no error)=w281) -> (error out=w298:errorcluster)
            n113 = Bundle By Name(cluster=w289, "Elements List"=w288) -> (w287:T6)
            n114 = property class="VI"(reference=w283, error in=w298, "FP.State"=T5."Standard" ("Front Panel Window:State")) -> (error out=w297:errorcluster)  [unwired: 1 out]
          }
          frame #1 {
          }
        }
      }
      frame #19 {
        # "Your code here.\n(You can make a copy of, or modify, this frame)"
        n115 = call <vilib>:"Add State(s) to Queue__jki_lib_state_machine.vi"("State(s) in (\"\")"=w307) -> ("States Out"=w306:string)  [unwired: 14 in]
      }
      frame #20 {
        # "Your code here.\n(You can make a copy of, or modify, this frame)"
        n116 = while {
          shift-right: [w323] -> w308
          shift-left: "Mail notification recipients" -> [w324]
          stop <- w320 stop-if-true
          n117 = Search 1D Array(1D array=w324, element="") -> (index of element=w322:i32)  [unwired: 1 in]
          n118 = Equal?(x=w322, y=-1) -> (x = y?=w320:bool)
          n119 = case shown="True" w320 {
            tunnel: w322 -> [w329 _]
            tunnel: w324 -> [w327 w330]
            tunnel: [w326 w330] -> w323
            frame #0 {
              n120 = Delete From Array(array=w327, length=1, index=w329) -> (array with subset deleted=w326:string[])  [unwired: 1 out]
            }
            frame #1 {
            }
          }
        }
        n121 = call <vilib>:"SMTP Email Send Message.vi"("recipients"=w308, "mail server"="smtp.lbl.gov", "return address"="ckoschitzki@lbl.gov", "subject ([No Subject])"="Automatic Laser Machining Message", "message"=w313, "error in (no error)"=w312) -> ("invalid recipients"=→"invalid recipients":string[], "error out"=w311:errorcluster)  [unwired: 8 in]
        n122 = call <vilib>:"Add State(s) to Queue__jki_lib_state_machine.vi"("State(s) in (\"\")"=w319) -> ("States Out"=w318:string)  [unwired: 14 in]
      }
      frame #21 {
        # "Template Separator\n(You can make a copy of, or modify, this frame)"
        n123 = call <vilib>:"Add State(s) to Queue__jki_lib_state_machine.vi"("State(s) in (\"\")"=w334) -> ("States Out"=w333:string)  [unwired: 14 in]
      }
      frame #22 {
        n124 = while {
          tunnel: [w405] -> w341
          stop <- w403 continue-if-true
          n125 = case shown="True" "Pause Machining" {
            frame #0 {
            }
            frame #1 {
              n126 = Wait (ms)(milliseconds to wait=u32 50) -> ()  [unwired: 1 out]
            }
          }
          n127 = Or(x="Pause Machining", y="Abort Machining") -> (x .or. y?=w403:bool)
          n128 = Not(x="Abort Machining") -> (.not. x?=w405:bool)
        }
        n129 = Unbundle By Name(w339) -> ("Current TRJ"=w343:i32, "TRJ Cluster.size(s)"=w346:i32, "Actual Element.Layer per L-Move"=w337:i32, "Actual Element.Element name"=w336:string)
        n130 = Less?(x=w343, y=w346) -> (x < y?=w345:bool)
        n131 = And(x=w345, y=w341) -> (x .and. y?=w344:bool)
        n132 = case shown="\"Demo\", Default" w335 {
          tunnel: w344 -> [w355 w388]
          tunnel: w343 -> [w354 w387]
          tunnel: [w353 w386] -> w342
          tunnel: [w352 w385] -> w340
          tunnel: w337 -> [w351 w384]
          tunnel: w336 -> [w350 w383]
          frame #0 {
            n133 = case shown="True" w355 {
              tunnel: w354 -> [w363 w367]
              tunnel: [w363 w375] -> w353
              tunnel: [w358 w369] -> w352
              tunnel: w351 -> [_ w368]
              tunnel: w350 -> [w360 _]
              frame #0 {
                w358 = "Machine:Close" ("State(s) in Front (\"\")")
                n134 = Concatenate Strings("Util:Mail>>" ("State(s) in Front (\"\")"), "The Element " ("string"), w360, " has finished machining!" ("string")) -> (w356:string)
                n135 = Concatenate Strings(w358, "\r\n", w356) -> ()  [unwired: 1 out]
              }
              frame #1 {
                n136 = Quotient & Remainder(x=w367, y=w368) -> (x-y*floor(x/y)=w366:i32)  [unwired: 1 out]
                n137 = Equal?(x=w366, y=0) -> (x = y?=w364:bool)
                n138 = case shown="True" w364 {
                  tunnel: ["" w378] -> w373
                  frame #0 {
                  }
                  frame #1 {
                    n139 = Number To Fractional String(number="Ablation Rate") -> (F-format string=w381:string)  [unwired: 3 in]
                    n140 = Concatenate Strings("\r\n", "Machine:MoveLens>>" ("State(s) in Front (\"\")"), w381) -> (w378:string)
                  }
                }
                n141 = Increment(x=w367) -> (x+1=w375:i32)
                n142 = Concatenate Strings("\r\n", "Machine:ExecMaster" ("State(s) in Front (\"\")")) -> (w370:string)
                n143 = Concatenate Strings("Machine:SetStartpoint\nMachine:Shutter>>Open\nMachine:ExecTRJ\nMachine:Shutter>>Close", w373, w370) -> (w369:string)
              }
            }
          }
          frame #1 {
            n144 = Wait (ms)(milliseconds to wait=u32 50) -> ()  [unwired: 1 out]
            n145 = case shown="True" w388 {
              tunnel: w387 -> [w394 w399]
              tunnel: [w394 w401] -> w386
              tunnel: [w389 "Machine:ExecMaster>>Demo" ("State(s) in Front (\"\")")] -> w385
              tunnel: w384 -> [_ w400]
              tunnel: w383 -> [w391 _]
              frame #0 {
                n146 = Concatenate Strings("Util:Mail>>" ("State(s) in Front (\"\")"), "The Element " ("string"), w391, " has finished machining!" ("string")) -> (w389:string)
              }
              frame #1 {
                n147 = Quotient & Remainder(x=w399, y=w400) -> (x-y*floor(x/y)=w398:i32)  [unwired: 1 out]
                n148 = Equal?(x=w398, y=0) -> (x = y?=→"Move Lens":bool)
                n149 = Increment(x=w399) -> (x+1=w401:i32)
              }
            }
          }
        }
        n150 = Bundle By Name(cluster=w339, "Current TRJ"=w342) -> (w338:T6)
        n151 = call <vilib>:"Add State(s) to Queue__jki_lib_state_machine.vi"("State(s) in (\"\")"=w349, "State(s) at Back (\"\")"=w340) -> ("States Out"=w348:string)  [unwired: 13 in]
      }
      frame #23 {
        w407 = u16 2 items=["Get Path", "Make Layout", "Create TRJs"] ("Outputmode")
        n152 = Unbundle By Name(w424) -> ("Elements available"=w419:T11, "Measured origin x,y"=w416:dbl[], "Actual Element"=w410:T8)  [unwired: 1 out]
        n153 = Unbundle By Name(w410) -> ("Type"=w414:i32)
        n154 = Index Array(array=w419, index=w414) -> (element=w411:T12)
        n155 = Unbundle By Name(w411) -> ("path"=w412:path)
        n156 = Open VI Reference(type specifier VI Refnum (for type only)=refnum<vi> refnum, vi path=w412, error in (no error)=w409) -> (vi reference=w422:refnum<vi>, error out=w418:errorcluster)  [unwired: 3 in]
        n157 = call "calc origin x0 y0.vi"("Measured origin x,y"=w416) -> ("Array"=w415:dbl[])
        n158 = property class="VI (strict)"(reference=w422, error in=w418, "Exec.ShowFPOnCall"=FALSE ("Execution:Show Front Panel On Call")) -> (reference out=w421:refnum<vi>, error out=w417:errorcluster)
        n159 = call-by-ref "Call By Reference Node"(reference=w421, error in=w417, "Measured origin x,y"=w415, "Element in"=w410, "Outputmode"=w407) -> (error out=w408:errorcluster, "TRJs"=w413:T13)  [unwired: 1 in, 4 out]
        n160 = Bundle By Name(cluster=w424, "TRJ Cluster"=w413) -> (w425:T6)
      }
      frame #24 {
        # "opens communication with xps and initialises stages if necessary"
        n161 = Unbundle By Name(w431) -> ("IP address"=w432:string, "Group Name"=w427:string)
        n162 = call <userlib>:"Open TCP-IP.vi"("error in (no error)"=w438, "IP address"=w432) -> ("error out"=w442:errorcluster, "Connection ID"=w443:T3)  [unwired: 4 in, 4 out]
        n163 = call <userlib>:"Open TCP-IP.vi"("error in (no error)"=w438, "IP address"=w432) -> ("error out"=w441:errorcluster, "Connection ID"=w440:T3)  [unwired: 4 in, 4 out]
        n164 = call <userlib>:"Firmware Version Get.vi"("error in (no error)"=w441, "connection ID in"=w440) -> ("error out"=w447:errorcluster, "XPS error out"=w448:errorcluster, "connection ID out"=w446:T3)  [unwired: 1 in, 6 out]
        n165 = call <userlib>:"Firmware Version Get.vi"("error in (no error)"=w442, "connection ID in"=w443) -> ("error out"=w451:errorcluster, "XPS error out"=w450:errorcluster, "connection ID out"=w449:T3)  [unwired: 1 in, 6 out]
        n166 = case shown="True" "Ture: Z home serch 2" {
          tunnel: [w457 w470] -> w444
          tunnel: [w456 w468] -> w445
          tunnel: [w455 w467] -> w436
          tunnel: w449 -> [w457 w466]
          tunnel: w450 -> [w456 w463]
          tunnel: w451 -> [w455 w462]
          frame #0 {
          }
          frame #1 {
            w469 = "S" ("Group Name 2")
            n167 = call <userlib>:"Group Kill.vi"("error in (no error)"=w462, "XPS error in (no error)"=w463, "Group Name (250 c max)"=w469, "connection ID in"=w466) -> ("error out"=w460:errorcluster, "XPS error out"=w461:errorcluster, "connection ID out"=w465:T3)  [unwired: 5 out]
            n168 = call <userlib>:"Group Initialize.vi"("error in (no error)"=w460, "XPS error in (no error)"=w461, "Group Name (250 c max)"=w469, "connection ID in"=w465) -> ("error out"=w458:errorcluster, "XPS error out"=w459:errorcluster, "connection ID out"=w464:T3)  [unwired: 5 out]
            n169 = call <userlib>:"Group Home Search.vi"("error in (no error)"=w458, "XPS error in (no error)"=w459, "Group Name (250 c max)"=w469, "connection ID in"=w464) -> ("error out"=w467:errorcluster, "XPS error out"=w468:errorcluster, "connection ID out"=w470:T3)  [unwired: 5 out]
          }
        }
        n170 = case shown="True" "Ture: XY home serch" {
          tunnel: [w473 w486] -> w430
          tunnel: [w472 w485] -> w428
          tunnel: [w471 w484] -> w437
          tunnel: w446 -> [w473 w483]
          tunnel: w447 -> [w471 w482]
          tunnel: w448 -> [w472 w477]
          tunnel: w427 -> [_ w474]
          frame #0 {
          }
          frame #1 {
            n171 = call <userlib>:"Group Kill.vi"("error in (no error)"=w482, "XPS error in (no error)"=w477, "Group Name (250 c max)"=w474, "connection ID in"=w483) -> ("error out"=w480:errorcluster, "XPS error out"=w476:errorcluster, "connection ID out"=w481:T3)  [unwired: 5 out]
            n172 = call <userlib>:"Group Initialize.vi"("error in (no error)"=w480, "XPS error in (no error)"=w476, "Group Name (250 c max)"=w474, "connection ID in"=w481) -> ("error out"=w478:errorcluster, "XPS error out"=w475:errorcluster, "connection ID out"=w479:T3)  [unwired: 5 out]
            n173 = call <userlib>:"Group Home Search.vi"("error in (no error)"=w478, "XPS error in (no error)"=w475, "Group Name (250 c max)"=w474, "connection ID in"=w479) -> ("error out"=w484:errorcluster, "XPS error out"=w485:errorcluster, "connection ID out"=w486:T3)  [unwired: 5 out]
          }
        }
        n174 = call <userlib>:"Single Axis Group Move Absolute.vi"("Target Position (units)"="Z Axis Position(S) (units)", "error in (no error)"=w436, "XPS error in (no error)"=w445, "SingleAxis Group  Name (250 c max)"="S", "connection ID in"=w444) -> ("error out"=w434:errorcluster)  [unwired: 6 out]
        n175 = Bundle By Name(cluster=w431, "connection ID"=w430, "XPS error"=w428) -> (w429:T6)
        n176 = call <vilib>:"Merge Errors.vi"("error in 2 (no error)"=w434, "error in 1 (no error)"=w437) -> ("error out"=w435:errorcluster)  [unwired: 5 in]
      }
      frame #25 {
        n177 = Fract/Exp String To Number(string=w492, offset=0, default (0 dbl)=0.0 ("default (0 I32)")) -> (number=w491:dbl)  [unwired: 1 in, 1 out]
        n178 = local read "connection ID out"() -> (w496:T3)
        n179 = local read "XPS error out"() -> (w499:errorcluster)
        n180 = call <userlib>:"Single Axis Group Move Relative.vi"("Target Displacement (units)"=w491, "error in (no error)"=w488, "XPS error in (no error)"=w499, "SingleAxis Group  Name (250 c max)"="SingleAxis Group  Name", "connection ID in"=w496) -> ("error out"=w487:errorcluster, "XPS error out"=w498:errorcluster, "connection ID out"=w497:T3)  [unwired: 4 out]
        n181 = local write "connection ID out"(w497) -> ()
        n182 = local write "XPS error out"(w498) -> ()
      }
      frame #26 {
        n183 = Unbundle By Name(w505) -> ("TRJ Cluster.TRJs"=w506:path[], "IP address"=w503:string)
        n184 = local read "XPS error out"() -> (w508:errorcluster)
        n185 = case shown="False" "Write to XPS" {
          tunnel: w508 -> [w510 w518]
          tunnel: [w510 w517] -> w507
          tunnel: w506 -> [_ w514]
          tunnel: w503 -> [_ w513]
          tunnel: w502 -> [w509 w512]
          tunnel: [w509 w511] -> w501
          frame #0 {
          }
          frame #1 {
            w515 = "Administrator" ("User")
            n186 = call "Multi_FTP_Put2.vi"("Address"=w513, "User"=w515, "Password"=w515, "trj file path 2"=w514, "XPS error in(no error)"=w518, "error in (no error)"=w512, "Cible Directory"="public\\trajectories") -> ("XPS error out"=w517:errorcluster, "error out"=w511:errorcluster)  [unwired: 7 in]
          }
        }
        "XPS error out(FTP put)" <- w507
        n187 = local write "XPS error out"(w507) -> ()
      }
      frame #27 {
        n188 = Unbundle By Name(w528) -> ("TRJ Cluster.Start Point"=w521:dbl[][], "Current TRJ"=w520:i32, "connection ID"=w523:T3, "XPS error"=w524:errorcluster, "Group Name"=w522:string)
        n189 = Index Array(array=w521, index (row)=w520) -> (element=w519:dbl[])  [unwired: 1 in]
        n190 = call <userlib>:"Axis Group Move Absolute.vi"("Target Position (units)"=w519, "error in (no error)"=w530, "XPS error in (no error)"=w524, "Group Name (250 c max)"=w522, "connection ID in"=w523) -> ("error out"=w529:errorcluster, "XPS error out"=w525:errorcluster, "connection ID out"=w526:T3)  [unwired: 4 out]
        n191 = Bundle By Name(cluster=w528, "connection ID"=w526, "XPS error"=w525) -> (w527:T6)
      }
      frame #28 {
        n192 = Unbundle By Name(w537) -> ("GPIO Name (DO)"=w543:string, "connection ID"=w542:T3, "XPS error"=w534:errorcluster)
        n193 = case shown="\"Close\", Default" w539 {
          tunnel: [0 ("Digital Output Value") 1 ("Digital Output Value")] -> w538
          frame #0 {
          }
          frame #1 {
          }
        }
        n194 = call <userlib>:"GPIO Digital Set.vi"("Digital Output Value"=w538, "Mask"=225, "error in (no error)"=w541, "XPS error in (no error)"=w534, "GPIO Name (DO)"=w543, "connection ID in"=w542) -> ("error out"=w540:errorcluster, "XPS error out"=w535:errorcluster, "connection ID out"=w536:T3)  [unwired: 3 out]
        n195 = Bundle By Name(cluster=w537, "connection ID"=w536, "XPS error"=w535) -> (w533:T6)
      }
      frame #29 {
        n196 = Unbundle By Name(w557) -> ("TRJ Cluster.TRJs"=w554:path[], "Current TRJ"=w552:i32, "connection ID"=w553:T3, "Group Name"=w548:string)  [unwired: 1 out]
        n197 = Index Array(array=w554, index=w552) -> (element=w551:path)
        n198 = local read "XPS error out"() -> (w559:errorcluster)
        n199 = Strip Path(path=w551) -> (name=w560:string)  [unwired: 1 out]
        n200 = call <userlib>:"XY Line Arc Verification.vi"("Trajectory File Name"=w560, "error in (no error)"=w550, "XPS error in (no error)"=w559, "XY Group Name (250 c max)"=w548, "connection ID in"=w553) -> ("error out"=w563:errorcluster, "XPS error out"=w562:errorcluster, "connection ID out"=w561:T3)  [unwired: 4 out]
        n201 = case shown="True" "Ture: execute trj" {
          tunnel: w548 -> [_ w577]
          tunnel: w562 -> [w567 w576]
          tunnel: w563 -> [w566 w575]
          tunnel: w561 -> [w568 w574]
          tunnel: [w568 w573] -> w556
          tunnel: [w567 w572] -> w564
          tunnel: [w566 w571] -> w549
          tunnel: "XY Line Arc Trajectory" -> [_ w570]
          tunnel: w560 -> [_ w569]
          frame #0 {
          }
          frame #1 {
            n202 = call <userlib>:"XY Line Arc Execution.vi"("XY Line Arc Trajectory"=w570, "Trajectory File Name"=w569, "error in (no error)"=w575, "XPS error in (no error)"=w576, "XY Group Name (250 c max)"=w577, "connection ID in"=w574) -> ("error out"=w571:errorcluster, "XPS error out"=w572:errorcluster, "connection ID out"=w573:T3)  [unwired: 3 out]
          }
        }
        n203 = local write "XPS error out"(w564) -> ()
        n204 = Bundle By Name(cluster=w557, "connection ID"=w556) -> (w555:T6)
      }
      frame #30 {
        n205 = Unbundle By Name(w578) -> ("connection ID"=w582:T3)
        n206 = call <userlib>:"Close TCP-IP.vi"("error in (no error)"=w581, "connection ID in"=w582) -> ("Error out"=w580:errorcluster)  [unwired: 9 out]
      }
      frame #31 {
        # "Template Separator\n(You can make a copy of, or modify, this frame)"
        n207 = call <vilib>:"Add State(s) to Queue__jki_lib_state_machine.vi"("State(s) in (\"\")"=w586) -> ("States Out"=w585:string)  [unwired: 14 in]
      }
    }
    "error out" <- w3
  }
  n208 = disable-structure shown="Disabled" {
    frame #0 {
      (unwired) "Data: Initialize\nInitialize Core Data\nUI: Initialize\nUI: Front Panel State >> Open"  # Data: Initialize Initialize Core Data UI: Initialize UI: Front Panel State >> Open
      n209 = Number To Decimal String(width (-)=i16 1) -> (decimal integer string=w589:string)  [unwired: 1 in]
      n210 = Concatenate Strings("CLayout:Main>>" ("State(s) in Front (\"\")"), w589) -> ()  [unwired: 1 out]
    }
    frame #1 {
    }
  }
